vi "nominal_channel_writer.write_data_cluster.vi"(8 "error in":errorcluster, 9 "Custom Cluster Streamer":refnum<class "stream_custom_cluster.lvclass">, 10 "Data Source RID":string, 11 "Nominal Client in":refnum<class "Nominal Client.lvclass">) -> (0 "error out":errorcluster, 2 "Response body":string, 3 "Nominal Client out":refnum<class "Nominal Client.lvclass">, 4 "Terminated":bool)   [LabVIEW 2020, in "Nominal Client.lvclass"]
doc: "Synchronously writes a data cluster of records to a Nominal data source.\n\nData Clusters must only contain scalar values (integers, floats, booleans, or strings). Nested clusters are allowed."
uses:
  Nominal Client.lvclass
  stream_custom_cluster/stream_custom_cluster.lvclass
  Nominal Client.lvclass/Nominal Client.ctl
  trace.payload_received.vi
  error.vi
  trace.payload_sent.vi
  create.authorization_header.vi
  trace.calling_method.vi
  error.vi/859f8e04-e495-489b-b5b4-7ac163f56130.vi
  <vilib>/JDP Science/JDP Science Common Utilities/Trim Whitespace__JDP.vi
  <vilib>/AdvancedString/1D String Array to Delimited String.vi
  api_token.get.vi
  <vilib>/Utility/libraryn.llb/Get File Extension.vi
  log_file.write.vi
  <vilib>/JDP Science/JSONtext/Get all Object Items.vi
  <vilib>/Utility/error.llb/Error Cluster From Error Code.vi
  <vilib>/JDP Science/JSONtext/JSON text to Variant.vi
  <vilib>/JDP Science/JSONtext/LVClass Serializer/JSONtext LVClass Serializer.lvclass
  <vilib>/addons/_JKI.lib/REST Client/classes/Response Headers/Response Headers.lvclass
  <vilib>/addons/_JKI.lib/REST Client/classes/REST Client/REST Client.lvclass
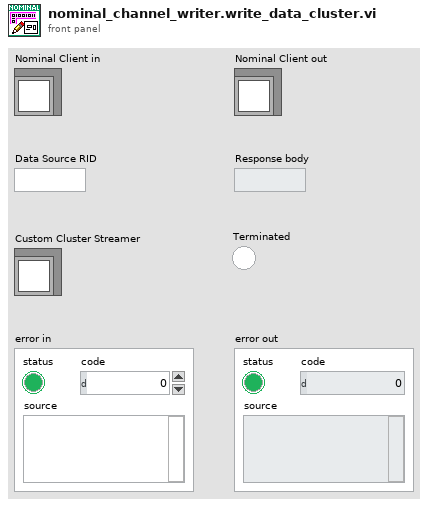
[diagram p1: front panel]
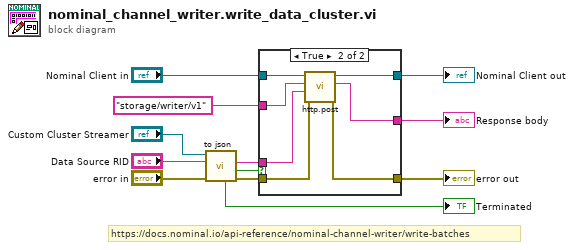
[diagram p0: block diagram]
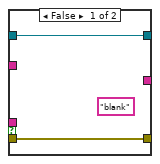
[diagram p2: hidden frame]
diagram:
  # "https://docs.nominal.io/api-reference/nominal-channel-writer/write-batches"
  n1 = call "to json.vi"("error in"="error in", "dataSourceRid"="Data Source RID", "stream_custom_cluster in"="Custom Cluster Streamer") -> ("error out"=w7:errorcluster, "Contains Data"=w2:bool, "json"=w3:string, "Terminated"=→"Terminated":bool)  [unwired: 4 in, 1 out]
  n2 = case shown="True" w2 {
    tunnel: "Nominal Client in" -> [w14 w21]
    tunnel: [w14 w20] -> w11
    tunnel: [w13 w19] -> w10
    tunnel: "storage/writer/v1" ("Path") -> [_ w18]
    tunnel: [_ w17] -> w8
    tunnel: w7 -> [w13 w16]
    tunnel: w3 -> [_ w15]
    frame False {
      (unwired) "blank" ("json")
    }
    frame True {
      n3 = call "http.post.vi"("error in"=w16, "Request body"=w15, "Path"=w18, "Nominal Client in"=w21) -> ("error out"=w19:errorcluster, "Response"=w17:string, "Nominal Client out"=w20:refnum<class "Nominal Client.lvclass">)  [unwired: 4 in, 1 out]
    }
  }
  "Nominal Client out" <- w11
  "error out" <- w10
  "Response body" <- w8
